vi "Read ch_alias.vi"(8 "error in (no error)":errorcluster, 11 "Sim DiscreteIO in":refnum<class "Sim DiscreteIO.lvclass">) -> (0 "error out":errorcluster, 2 "ch_alias":string[](array[string]), 3 "Sim DiscreteIO out":refnum<class "Sim DiscreteIO.lvclass">)   [LabVIEW 2021, in "Sim DiscreteIO.lvclass"]
uses:
  Sim DiscreteIO.lvclass
  Sim DiscreteIO.lvclass/Sim DiscreteIO.ctl
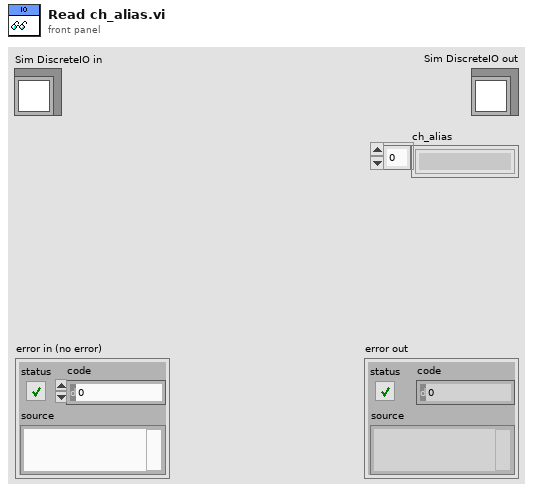
[diagram p1: front panel]
types:
  T1 = typedef "Sim DiscreteIO.lvclass/DVR.ctl" = cluster{"ch_labels":string[], "_PARMS":T2, "Initialized?":bool, "occurrence":refnum<k4>}
  T2 = typedef "Sim DiscreteIO.lvclass/_PARMS.ctl" = cluster{"ch_units":string[], "ch_alias":string[]}
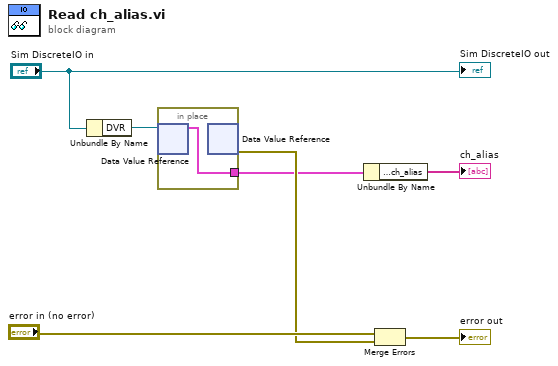
[diagram p0: block diagram]
diagram:
  n1 = Unbundle By Name ("DVR Unbundle")("Sim DiscreteIO in") -> ("DVR"=w3:refnum<data-value>)
  n2 = in-place "In Place Element Structure" {
    in-place-border: [w8] -> w2
    n3 = in-place-dvr #1(w3) -> (w8:T1)  [unwired: 1 out]
    n4 = in-place-dvr #1() -> (w4:errorcluster)  [unwired: 1 in, 1 out]
  }
  n5 = Unbundle By Name ("Item Unbundle")(w2) -> ("_PARMS.ch_alias"=→"ch_alias":string[])
  n6 = Merge Errors("error in (no error)", w4) -> (→"error out":errorcluster)
  "Sim DiscreteIO out" <- "Sim DiscreteIO in"
